vi "Gen Stage 4 Update Supporting Projects.vi"(7 "Staus":refnum<vi>, 8 "error in (no error)":errorcluster, 10 "New Name":string, 11 "Template Project Path":path) -> (0 "error out":errorcluster)   [LabVIEW 2021, in "Plugin Generator.lvlib"]
uses:
  Plugin Generator.lvlib
  <vilib>/CIF Foundation/CIF LabVIEW Scripting/LV Scripting/LV Scripting Utilities.lvlib
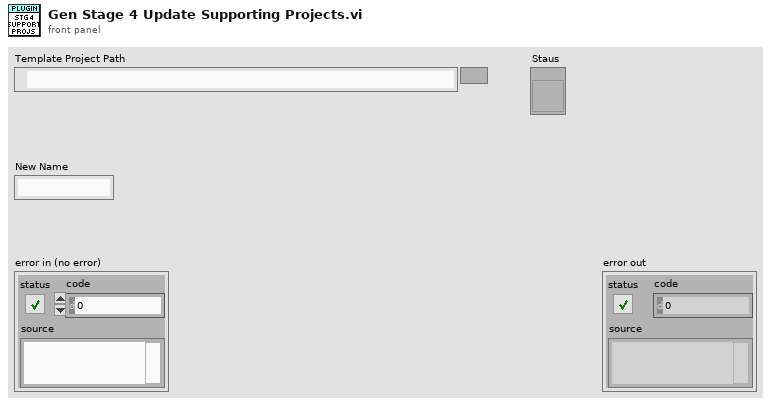
[diagram p1: front panel]
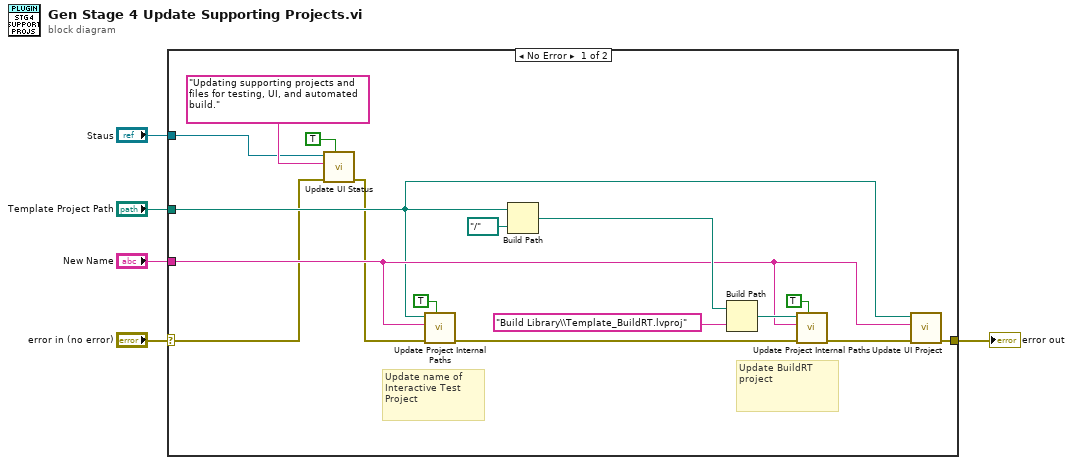
[diagram p0: block diagram]
diagram:
  n1 = case shown="No Error" "error in (no error)" {
    selector: "error in (no error)" -> [w7 w22]
    tunnel: "New Name" -> [w14 _]
    tunnel: "Template Project Path" -> [w13 _]
    tunnel: [w12 w22] -> w3
    tunnel: "Staus" -> [w9 _]
    frame No Error {
      # "Update BuildRT project"
      # "Update name of Interactive Test Project"
      n2 = call "Update UI Status.vi"("Previous Complete"=TRUE, "error in"=w7, "Status to Display"="Updating supporting projects and files for testing, UI, and automated build." ("To display"), "String in"=w9) -> ("error out"=w8:errorcluster)  [unwired: 7 in]
      n3 = call <vilib>:"Update Project Internal Paths.vi"("Rename Project"=TRUE, "error in (no error)"=w8, "New Subname"=w14, "Project Path"=w13) -> ("error out"=w11:errorcluster)  [unwired: 7 in]
      n4 = Build Path(base path=w13, name or relative path=path "../..") -> (appended path=w17:path)
      n5 = Build Path(base path=w17, name or relative path="Build Library\\Template_BuildRT.lvproj" ("Class Name")) -> (appended path=w19:path)
      n6 = call <vilib>:"Update Project Internal Paths.vi"("Rename Project"=TRUE, "error in (no error)"=w11, "New Subname"=w14, "Project Path"=w19) -> ("error out"=w15:errorcluster)  [unwired: 7 in]
      n7 = call "Update UI Project.vi"("error in (no error)"=w15, "New Name"=w14, "Template Project Path"=w13) -> ("error out"=w12:errorcluster)  [unwired: 8 in]
    }
    frame Error {
    }
  }
  "error out" <- w3
